vi "save operation.vi"(7 "force save as":bool, 8 "error in":errorcluster, 11 "state cluster":T1) -> (0 "error out":errorcluster, 3 "state out":T1)   [LabVIEW 2013, in "RT Temperature Controller.lvlib"]
uses:
  RT Temperature Controller.lvlib
  Controls/StateCluster.ctl
  <vilib>/NI/Tag Bus Data Framework/Configuration Editor/Classes/SystemConfigRepo/SystemConfigRepo.lvclass
  <vilib>/CEF_TreeControl/Node/NodeRef.ctl
  <vilib>/CEF_TreeControl/Node/NISE_CEF_Node.lvclass
  <vilib>/CEF_TreeControl/Node/UserEventRef.ctl
  <vilib>/CEF_TreeControl/Controls/EventCluster.ctl
  SplashScreen/splash screen.ctl
  SplashScreen/notifier data.ctl
  <vilib>/CEF_TreeControl/NISE_CEF_TreeControl.lvlib
  SplashScreen/splash screen.lvlib
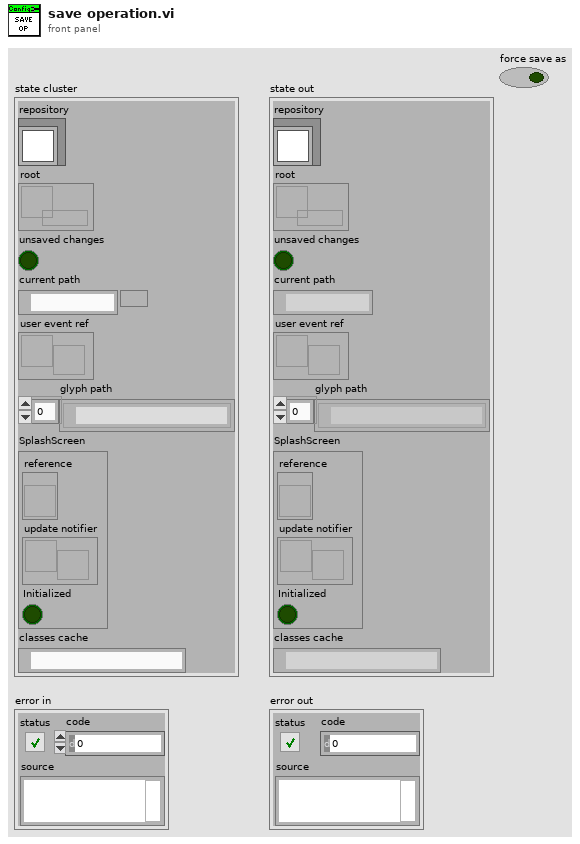
[diagram p1: front panel]
types:
  T1 = typedef "RT Temperature Controller.lvlib/StateCluster.ctl" = cluster{"repository":refnum<class "SystemConfigRepo.lvclass">, "root":T2, "unsaved changes":bool, "current path":path, "user event ref":T3, "glyph path":path[], "SplashScreen":T4, "classes cache":path}
  T2 = typedef "NISE_CEF_Node.lvclass/NodeRef.ctl" = refnum<data-value>
  T3 = typedef "NISE_CEF_Node.lvclass/UserEventRef.ctl" = refnum<user-event>
  T4 = typedef "RT Temperature Controller.lvlib/splash screen.lvlib/splash screen.ctl" = cluster{"reference":refnum<vi>, "update notifier":refnum<notifier>, "Initialized":bool}
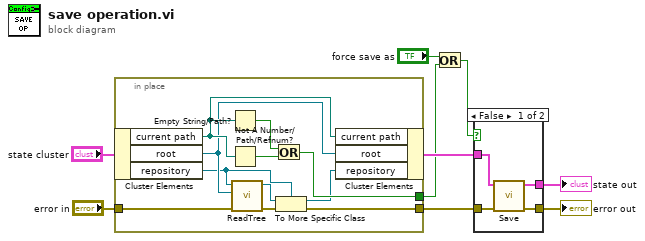
[diagram p0: block diagram]
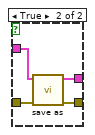
[diagram p2: hidden frame]
diagram:
  n1 = in-place {
    in-place-border: [w17] -> w3
    in-place-border: "error in" -> [w16]
    in-place-border: [w13] -> w9
    n2 = in-place-cluster #1("state cluster") -> ("current path"=w18:path, "root"=w15:T2, "repository"=w11:refnum<class "SystemConfigRepo.lvclass">)
    n3 = Empty String/Path?(string/path=w18) -> (empty?=w19:bool)
    n4 = Not A Number/Path/Refnum?(number/path/refnum=w18) -> (NaN/Path/Refnum?=w20:bool)
    n5 = call-dynamic "ReadTree.vi"("error in"=w16, "root"=w15, "SystemConfigRepo in"=w11) -> ("error out"=w14:errorcluster, "repository out"=w12:refnum<class "NISE_CEF_Repository.lvclass">)  [unwired: 7 in]
    n6 = Or(x=w19, y=w20) -> (x .or. y?=w17:bool)
    n7 = To More Specific Class(target class=w11, reference=w12, error in=w14) -> (specific class reference=w10:refnum<class "SystemConfigRepo.lvclass">, error out=w13:errorcluster)
    n8 = in-place-cluster #1("current path"=w18, "root"=w15, "repository"=w10) -> (w8:T1)
  }
  n9 = Or(x="force save as", y=w3) -> (x .or. y?=w2:bool)
  n10 = case shown="False" w2 {
    tunnel: w8 -> [w24 w26]
    tunnel: [w23 w25] -> w4
    tunnel: [w22 w27] -> w7
    tunnel: w9 -> [w21 w28]
    frame False {
      n11 = call "Save.vi"("error in"=w21, "state in"=w24) -> ("error out"=w22:errorcluster, "state out"=w23:T1)  [unwired: 8 in]
    }
    frame True {
      n12 = call "save as.vi"("error in"=w28, "state in"=w26) -> ("error out"=w27:errorcluster, "state out"=w25:T1)  [unwired: 7 in, 1 out]
    }
  }
  "error out" <- w7
  "state out" <- w4
